vi "Write Report.vi"(8 "error in (no error)":errorcluster, 10 "Resource In":variant, 11 "Analyze Parameter Calibration in":refnum<class "Analyze Parameter Calibration.lvclass">) -> (0 "error out":errorcluster, 2 "Resource Out":variant, 3 "Analyze Parameter Calibration out":refnum<class "Analyze Parameter Calibration.lvclass">)   [LabVIEW 2020, in "Analyze Parameter Calibration.lvclass"]
uses:
  Analyze Parameter Calibration.lvclass
  C:/POLARIS Programme/POLARIS-AS-3-Cams/Submodules/HIJ Vision/Analyze/Analyze Parameter/Analyze Parameter Base/Analyze Parameter Base.lvclass
  <vilib>/Utility/config.llb/Config Data RefNum.ctl
  Analyze Parameter Calibration.lvclass/Analyze Parameter Calibration.ctl
  <vilib>/Utility/config.llb/Write Key (Double).vi
  <vilib>/Utility/config.llb/NI_LVConfig.lvlib
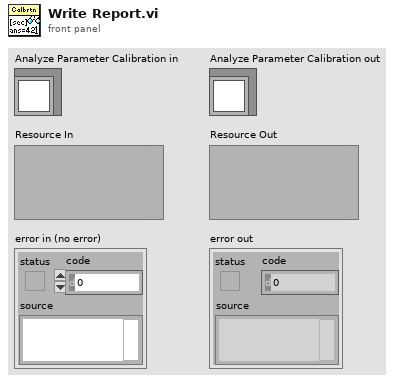
[diagram p1: front panel]
types:
  T1 = typedef "NI_LVConfig.lvlib/Config Data RefNum.ctl" = refnum<k1>
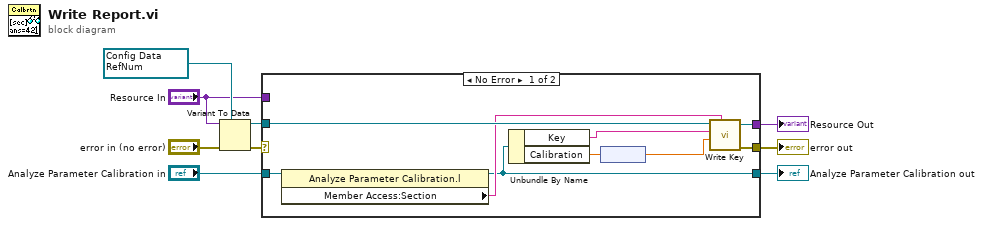
[diagram p0: block diagram]
diagram:
  w9 = T1 refnum items=["config data"] ("refnum")
  n1 = Variant To Data(error in="error in (no error)", type=w9, Variant="Resource In") -> (data=w8:T1, error out=w2:errorcluster)
  n2 = case shown="No Error" w2 {
    selector: w2 -> [_ w20]
    tunnel: w8 -> [w18 _]
    tunnel: "Analyze Parameter Calibration in" -> [w17 w19]
    tunnel: [w13 w19] -> w6
    tunnel: [w15 w21] -> w5
    tunnel: [w14 w20] -> w3
    tunnel: "Resource In" -> [_ w21]
    frame No Error {
      n3 = property class="Analyze Parameter Calibration.l"(reference=w17) -> (reference out=w13:refnum<class "Analyze Parameter Calibration.lvclass">, "Member Access:Section"=w16:string)  [unwired: 1 in, 1 out]
      n4 = Unbundle By Name(w13) -> ("Key"=w12:string, "Calibration"=w11:dbl[unit])
      n5 = node(w11) -> (w10:dbl)
      n6 = call-poly <vilib>:"Write Key.vi"("section"=w16, "value"=w10, "key"=w12, "refnum"=w18) -> ("error out"=w14:errorcluster, "refnum out"=w15:T1)  [unwired: 5 in, 1 out]
    }
    frame Error {
    }
  }
  "error out" <- w3
  "Analyze Parameter Calibration out" <- w6
  "Resource Out" <- w5
